vi "Motor Control Loop.vi"(8 "error in":errorcluster) -> (0 "error out":errorcluster)   [LabVIEW 2011]
uses:
  <vilib>/Simulation/Scripting/Companion Diagram/SimConfigNode/SimParams.ctl
  <vilib>/Simulation/Scripting/Companion Diagram/SimConfigNode/_simSolvers.ctl
  <vilib>/Simulation/Implementation/Shared/SIMSCR Execution Mode.ctl
  <vilib>/Platform/TimedLoop/XDataNode/timing_clust.ctl
  <vilib>/Platform/TimedLoop/XDataNode/nitl_modes.ctl
  <vilib>/Platform/TimedLoop/XDataNode/wakeup.ctl
  <vilib>/Simulation/Param Hierarchy/Typedefs/SIMPH Param Control Actions.ctl
  <vilib>/Simulation/Implementation/Shared/SIM limit type.ctl
  <vilib>/Simulation/Implementation/Shared/NILVSim_FinishedLate.vi
  <vilib>/Simulation/Utility/Implementation/SIM Halt.vi
  <vilib>/Simulation/Nonlinear/Implementation/NILVSim Saturation.llb/SIM Saturation (vector).vi
  <vilib>/Simulation/Nonlinear/Implementation/NILVSim Saturation.llb/SIM Saturation (scalar).vi
  <vilib>/Simulation/ContinuousLinear/Implementation/NILVSim Integrator new.llb/SIM Integrator distributor (scalar).vi
  <vilib>/Simulation/ContinuousLinear/Implementation/NILVSim Integrator new.llb/SIM Integrator collector (scalar).vi
  <vilib>/Simulation/ContinuousLinear/Implementation/NILVSim Integrator new.llb/SIM Integrator Collector (vector).vi
  <vilib>/Simulation/ContinuousLinear/Implementation/NILVSim Integrator new.llb/SIM Integrator Distributor (vector).vi
  <vilib>/Simulation/Implementation/Shared/SIM Is Init or Final Stage.vi
  <vilib>/Simulation/Implementation/Shared/NILVSim_Manager.vi
  <vilib>/Simulation/Implementation/Shared/NILVSim_ParamChanged.vi
  <vilib>/Simulation/Implementation/Shared/NILVSim_FinalizeModel.vi
  Robot Parameters/Robot Parameters.vi
  Roboteq/Public/Set RPM.vi
  <vilib>/Simulation/Implementation/Shared/SIM Unbundle Sim Info.vi
  <vilib>/Simulation/Implementation/Shared/NILVSim_GetModelError.vi
  <vilib>/Simulation/Implementation/Shared/SIM Bundle Sim Info.vi
  <vilib>/Simulation/Implementation/Shared/NILVSim_Initialize.vi
  <vilib>/robotics/Steering/Steering Frame/Apply Velocity to Motors.vi
  <vilib>/robotics/Steering/Steering Frame/Apply Steering Frame Velocity to Motors.vi
  Unsaturate Commanded Motor Velocities.vi
  <vilib>/robotics/Steering/Steering Frame/Get Velocity from Motors.vi
  <vilib>/robotics/Steering/Steering Frame/Get Steering Frame Velocity from Motors.vi
  <vilib>/Analysis/coordinate.llb/2D Cartesian Coordinate Rotation.vi
  <vilib>/Analysis/coordinate.llb/2D Cartesian Coordinate Rotation (Scalar).vi
  <vilib>/Simulation/Scripting/Companion Diagram/SimConfigNode/SimDog.xnode
  <vilib>/Platform/TimedLoop/XDataNode/XDataNode.xnode
  <vilib>/Simulation/Model Libraries/PID/SIM PID (Parallel).vi
  <vilib>/Simulation/Model Libraries/PID/SIM PID.vi
  <vilib>/Simulation/Implementation/XNodeFramework/SimXNode/SimX.xnode
  <vilib>/Platform/TimedLoop/XDataNode/XDNodeRunTimeDep.lvlib
  Roboteq/Roboteq.lvlib
  <vilib>/robotics/Steering/Steering Frame/NI_Robotics_Steering Frame.lvclass
  <vilib>/Analysis/NI_AALPro.lvlib
  <vilib>/Simulation/ContinuousLinear/Implementation/NILVSim Integrator new.llb/SIM Integrator (vector).vi
  <vilib>/Simulation/ContinuousLinear/Implementation/NILVSim Integrator new.llb/SIM Integrator (scalar).vi
  <vilib>/robotics/Utilities/NI_Robotics Utilities.lvlib
  <vilib>/Simulation/Implementation/Shared/NI_SIM_Implementation.lvlib
panel:
  out "Telemetry":T1={"Voltage"={0.0, 0.0, 0.0}, "Encoder Speed"={0, 0}, "Temps"={"IC Temp (C)"=0, "Ch1 Temp (C)"=0, "Ch2 Temp (C)"=0}, "Current"={0.0, 0.0, 0.0, 4.6238981750249924e+36}} {"Current" scale=0.0..16.0; "Temps"."IC Temp (C)" scale=0.0..150.0; "Temps"."Ch1 Temp (C)" scale=0.0..150.0; "Temps"."Ch2 Temp (C)" scale=0.0..150.0; "Encoder Speed" scale=-100.0..100.0; "Voltage" scale=8.0..14.0}
  in  "VISA resource name":refnum<visa-resource-name>
  in  "Debug":bool
  out "Command to Serial":string
  in  "End Loop":bool
  in  "stop?":bool
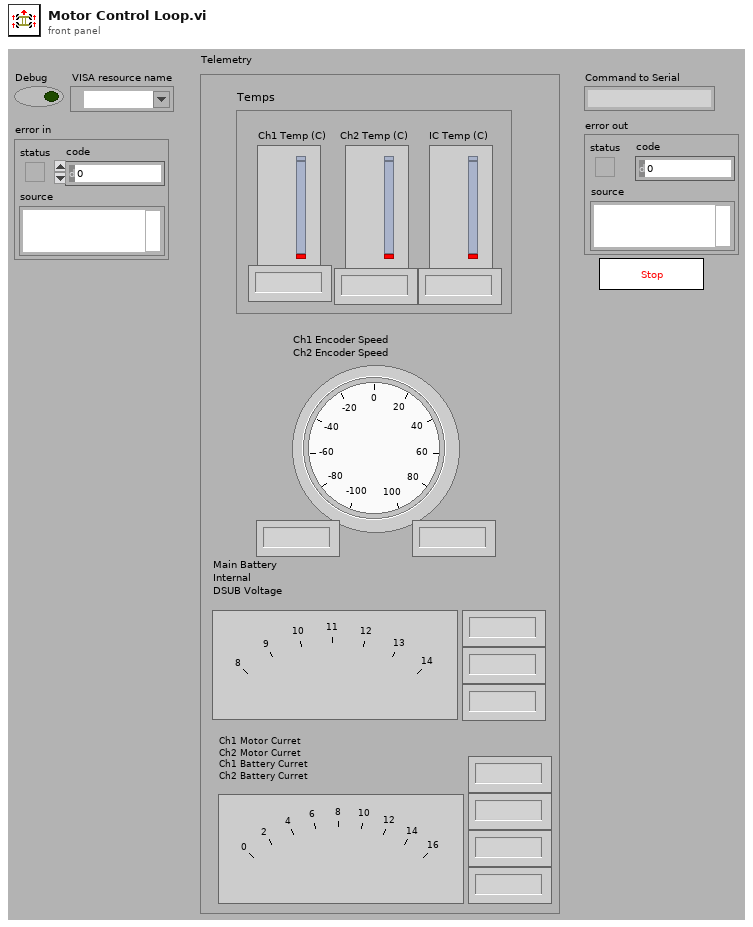
[diagram p1: front panel]
types:
  T1 = cluster{"Voltage":cluster{sgl, sgl, sgl}, "Encoder Speed":cluster{i32, i32}, "Temps":cluster{"IC Temp (C)":i32, "Ch1 Temp (C)":i32, "Ch2 Temp (C)":i32}, "Current":cluster{dbl, dbl, dbl, dbl}}
  T2 = typedef "SIMPH Param Control Actions.ctl" = enum16{"get params", "set params"}
  T3 = typedef "SIM limit type.ctl" = enum16{"upper", "lower", "both", "none"}
  T4 = typedef "XDNodeRunTimeDep.lvlib/timing_clust.ctl" = cluster{"Expected End [f-1]":u64, "Actual End [f-1]":u64, "Finished Late? [f-1]":bool, "Expected End [i-1]":u64, "Actual End [i-1]":u64, "Finished Late? [i-1]":bool, "Expected Start [i]":u64, "Actual Start [i]":u64, "Expected Start [f]":u64, "Actual Start [f]":u64, "Source Name":string, "Structure Name":string, "Period":i64, "Deadline":i64, "Offset":i64, "Start":i64, "Priority":i32, "Timeout":i32, "Mode":T5, "Wakeup Reason":T6, "Error":errorcluster, "Source Type":string, "Secondary Source Type":string, "Global End Time":u64, "Global Start Time":u64, "Frame Duration":u64, "Iteration Duration":u64, "Assigned CPU":i32, "I/O Scan Engine Mode":u32}
  T5 = typedef "XDNodeRunTimeDep.lvlib/nitl_modes.ctl" = enum32{"No Change", "Process missed periods, maintain original phase", "Discard missed periods, maintain original phase", "Process missed periods, ignore original phase", "Discard missed periods, ignore original phase"}
  T6 = typedef "XDNodeRunTimeDep.lvlib/wakeup.ctl" = enum32{"Normal", "Aborted", "Asynchronous wakeup", "Timing source error", "Timed loop error", "Timeout"}
  T7 = typedef "SimParams.ctl" = cluster{"Initial Time (s)":dbl, "Final Time (s)":dbl, "Step Size (s)":dbl, "ODE Solver":T8, "Minimum Step Size (s)":dbl, "Maximum Step Size (s)":dbl, "Relative Tolerance":dbl, "Absolute Tolerance":dbl, "Software Timing":bool, "Initial Step Size (s)":dbl, "Automatic Fixed Step Size?":bool, "Automatic Discrete Step Size?":bool, "Discrete Step Size (s)":dbl, "Calculate using Time Step":bool, "Solver Wired?":bool, "Prev.Frm.Expected End":u64, "Prev.Frm.Actual End":u64, "Prev.Frm.Finished Late?":bool, "Prev.Iter.Expected End":u64, "Prev.Iter.Actual End":u64, "Prev.Iter.Finished Late?":bool, "Expected Iteration Start":u64, "Actual Iteration Start":u64, "Expected Frame Start":u64, "Actual Frame Start":u64, "Source Name":string, "Name":string, "Period":i64, "Deadline":i64, "Offset":i64, "Start":i64, "Priority":i32, "Timeout":i32, "Processor":i32, "Mode":enum32{"No Change", "Process missed periods, maintain original phase", "Discard missed periods, maintain original phase", "Process missed periods, ignore original phase", "Discard missed periods, ignore original phase"}, "Wakeup reason":enum32{"Normal", "Aborted", "Asynchronous wakeup", "Timing source error", "Timed loop error", "Timeout"}, "Error":errorcluster, "Source Type":string, "Secondary Source Type":string, "Global End Time":u64, "Global Start Time":u64, "Full Solver Reset":bool, "Execution Mode":T9, "Nan/Inf Check":bool, "Custom Solver Library":string, "Solver Is Variable":bool, "custom solver name":string}
  T8 = typedef "_simSolvers.ctl" = enum16{"Runge-Kutta 1 (Euler)", "Runge-Kutta 2", "Runge-Kutta 3", "Runge-Kutta 4", "Runge-Kutta 23 (variable)", "Runge-Kutta 45 (variable)", "BDF (variable)", "Adams-Moulton (variable)", "Rosenbrock (variable)", "Discrete States Only", "Linearizer", "State Query", "Trim Eval", "Custom Solver"}
  T9 = typedef "SIMSCR Execution Mode.ctl" = u16
  T10 = cluster{"main battery voltage (V)":sgl, "internal voltage (V)":sgl, "DSUB voltage (V)":sgl}
  T11 = cluster{" Ch1  Motor current (I)":sgl, " Ch2 Motor current (I)":sgl, " Ch1 Battery current (I)":sgl, " Ch2 Battery current (I)":sgl}
  T12 = cluster{"Ch1 Temp (C)":i32, "Ch2 Temp (C)":i32, "IC Temp (C)":i32}
  T13 = cluster{"Encoder Speed (RPM)":i32, "Encoder Speed (RPM)":i32}
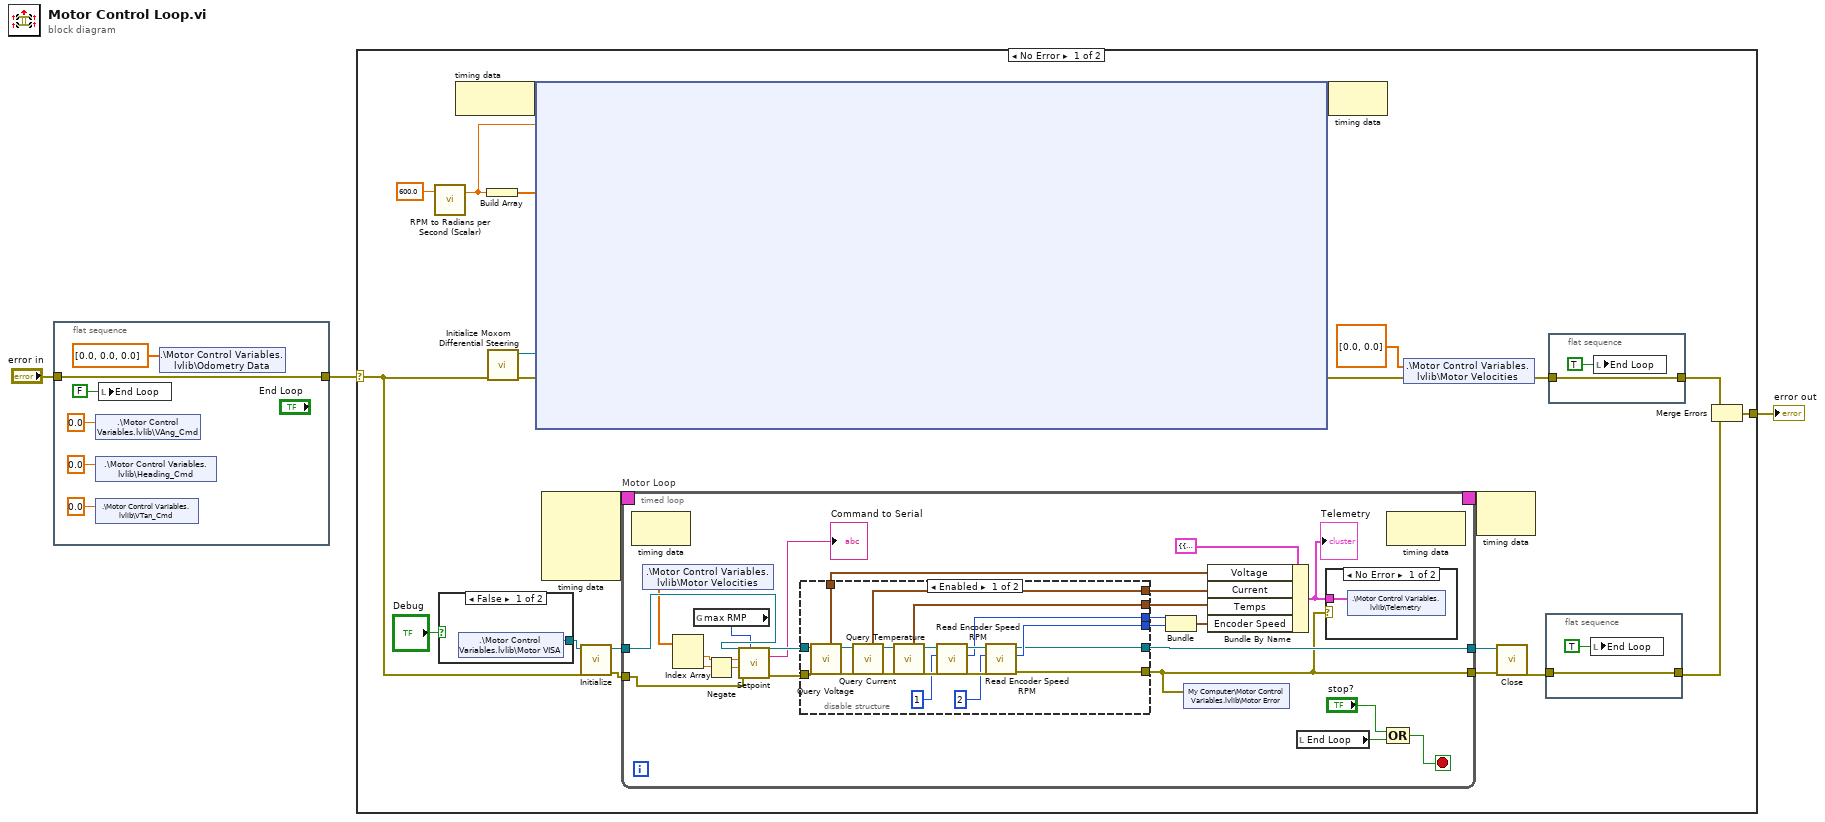
[diagram p0: block diagram]
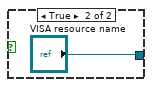
[diagram p2: hidden frame]
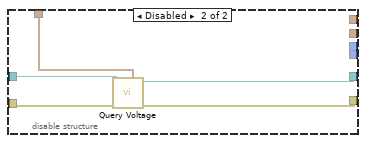
[diagram p3: hidden frame]
diagram:
  n1 = flat-sequence {
    tunnel: [w5] -> w2
    tunnel: "error in" -> [w5]
    frame #0 {
      n2 = shared-variable ".\\Motor Control Variables.lvlib\\VAng_Cmd"(0.0 ("VX_Cmd")) -> ()  [unwired: 1 in, 1 out]
      n3 = shared-variable ".\\Motor Control Variables.lvlib\\Heading_Cmd"(0.0 ("Heading_Cmd")) -> ()  [unwired: 1 in, 1 out]
      n4 = shared-variable ".\\Motor Control Variables.lvlib\\VTan_Cmd"(0.0 ("VY_Cmd")) -> ()  [unwired: 1 in, 1 out]
      n5 = local write "End Loop"(FALSE ("End Loop")) -> ()
      n6 = shared-variable ".\\Motor Control Variables.lvlib\\Odometry Data"(dbl[] [0.0, 0.0, 0.0] ("Odometry Data")) -> ()  [unwired: 1 in, 1 out]
    }
  }
  n7 = case shown="No Error" w2 {
    selector: w2 -> [w28 w495]
    tunnel: [w30 w495] -> w1
    frame No Error {
      n8 = call <vilib>:"RPM to Radians per Second (Scalar).vi"("rpm"=600.0 ("Numeric")) -> ("radians per second"=w16:dbl)  [unwired: 2 in]
      n9 = case shown="False" "Debug" {
        tunnel: [w33 "VISA resource name"] -> w29
        frame False {
          n10 = shared-variable ".\\Motor Control Variables.lvlib\\Motor VISA"() -> (w33:refnum<visa-resource-name>)  [unwired: 1 in, 1 out]
        }
        frame True {
        }
      }
      n11 = node-c288() -> (w18:variant)  [unwired: 1 in]
      n12 = Build Array(w16) -> (w15:dbl[])
      n13 = call "Initialize Moxom Differential Steering.vi"("error in (no error)"=w28) -> ("error out"=w12:errorcluster, "differential steering frame out"=w13:refnum<class "NI_Robotics_Differential Steering Frame.lvclass">)  [unwired: 9 in]
      n14 = node-c254 ("Simulation Loop 3")(w18, w16, w15, w12, w13) -> (w17:variant, w11:errorcluster)
      n15 = node-c288() -> (w20:T4)  [unwired: 4 in]
      n16 = call "Initialize.vi"("error in (no error)"=w28, "VISA resource name"=w29) -> ("error out"=w26:errorcluster, "VISA resource name out"=w27:refnum<visa-resource-name>)  [unwired: 8 in]
      n17 = timed-loop "Motor Loop" {
        tunnel: w27 -> [w459]
        tunnel: w26 -> [w458]
        tunnel: [w453] -> w25
        tunnel: [w454] -> w31
        timing: w20 -> [_]
        timing-out: [_] -> w19
        stop <- w460 stop-if-true
        n18 = node-c288() -> ()  [unwired: 1 in, 1 out]
        n19 = shared-variable ".\\Motor Control Variables.lvlib\\Motor Velocities"() -> (w441:dbl[])  [unwired: 1 in, 1 out]
        n20 = Index Array(array=w441) -> (element #1=w449:dbl, element #2=w442:dbl)  [unwired: 2 in]
        n21 = global read "Robot Parameters.vi" "max RMP"() -> (w450:i32)
        n22 = Negate(x=w442) -> (-x=w439:dbl)
        n23 = call-poly "Setpoint.vi"("Max RPM"=w450, "error in (no error)"=w458, "Motor2 Speed (RPM)"=w439, "Motor1 Speed (RPM)"=w449, "VISA resource name"=w459) -> ("error out"=w455:errorcluster, "Command"=→"Command to Serial":string, "VISA resource name out"=w456:refnum<visa-resource-name>)  [unwired: 4 in]
        n24 = disable-structure shown="Enabled" {
          disable-tunnel: w456 -> [w480 w485]
          disable-tunnel: w455 -> [w479 w484]
          disable-tunnel: [w474 _] -> w445
          disable-tunnel: [w473 _] -> w444
          disable-tunnel: [w463 w483] -> w454
          disable-tunnel: [w472 _] -> w446
          disable-tunnel: [w462 w482] -> w453
          disable-tunnel: [w471 w481] -> w447
          disable-tunnel: [w466 _] -> w440
          frame Enabled {
            n25 = call "Query Voltage.vi"("error in (no error)"=w479, "VISA resource name"=w480) -> ("error out"=w469:errorcluster, "VISA resource name out"=w470:refnum<visa-resource-name>, "Voltages"=w471:T10)  [unwired: 4 in, 3 out]
            n26 = call "Query Current.vi"("error in (no error)"=w469, "VISA resource name"=w470) -> ("error out"=w467:errorcluster, "VISA resource name out"=w468:refnum<visa-resource-name>, "Motor Currents"=w466:T11)  [unwired: 3 in, 4 out]
            n27 = call "Query Temperature.vi"("error in (no error)"=w467, "VISA resource name"=w468) -> ("error out"=w477:errorcluster, "VISA resource name out"=w478:refnum<visa-resource-name>, "Temps"=w472:T12)  [unwired: 4 in, 3 out]
            n28 = call "Read Encoder Speed RPM.vi"("error in (no error)"=w477, "channel number"=u8 1, "VISA resource name"=w478) -> ("error out"=w475:errorcluster, "Encoder Speed (RPM)"=w474:i32, "VISA resource name out"=w476:refnum<visa-resource-name>)  [unwired: 6 in]
            n29 = call "Read Encoder Speed RPM.vi"("error in (no error)"=w475, "channel number"=u8 2, "VISA resource name"=w476) -> ("error out"=w462:errorcluster, "Encoder Speed (RPM)"=w473:i32, "VISA resource name out"=w463:refnum<visa-resource-name>)  [unwired: 6 in]
          }
          frame Disabled {
            n30 = call "Query Voltage.vi"("error in (no error)"=w484, "VISA resource name"=w485) -> ("error out"=w482:errorcluster, "VISA resource name out"=w483:refnum<visa-resource-name>, "Voltages"=w481:T10)  [unwired: 4 in, 3 out]
          }
        }
        n31 = Bundle("Encoder Speed (RPM)"=w445, "Encoder Speed (RPM)"=w444) -> (w443:T13)  [unwired: 1 in]
        n32 = shared-variable "My Computer\\Motor Control Variables.lvlib\\Motor Error"(w453) -> ()  [unwired: 1 in, 1 out]
        n33 = Bundle By Name(cluster=T1 {"Voltage"={0.0, 0.0, 0.0}, "Encoder Speed"={0, 0}, "Temps"={"IC Temp (C)"=0, "Ch1 Temp (C)"=0, "Ch2 Temp (C)"=0}, "Current"={0.0, 0.0, 0.0, 0.0}} ("Telemetry"), "Voltage"=w447, "Current"=w440, "Temps"=w446, "Encoder Speed"=w443) -> (w451:T1)
        "Telemetry" <- w451
        n34 = local read "End Loop"() -> (w457:bool)
        n35 = case shown="No Error" w453 {
          tunnel: w451 -> [w488 _]
          frame No Error {
            n36 = shared-variable ".\\Motor Control Variables.lvlib\\Telemetry"(w488) -> ()  [unwired: 1 in, 1 out]
          }
          frame Error {
          }
        }
        n37 = node-c288() -> ()  [unwired: 1 in, 1 out]
        n38 = Compound Arithmetic op=OR("stop?", w457) -> (w460:bool)
      }
      n39 = node-c288(w17) -> ()  [unwired: 1 out]
      n40 = shared-variable ".\\Motor Control Variables.lvlib\\Motor Velocities"(dbl[] [0.0, 0.0] ("Motor Velocities"), error in=w11) -> (error out=w21:errorcluster)
      n41 = node-c288(w19) -> ()  [unwired: 1 out]
      n42 = call "Close.vi"("error in (no error)"=w25, "VISA resource name"=w31) -> ("error out"=w24:errorcluster)  [unwired: 9 in]
      n43 = flat-sequence {
        tunnel: w24 -> [w491]
        tunnel: [w491] -> w23
        frame #0 {
          n44 = local write "End Loop"(TRUE ("End Loop")) -> ()
        }
      }
      n45 = flat-sequence {
        tunnel: [w493] -> w22
        tunnel: w21 -> [w493]
        frame #0 {
          n46 = local write "End Loop"(TRUE ("End Loop")) -> ()
        }
      }
      n47 = Merge Errors(w22, w23) -> (w30:errorcluster)
    }
    frame Error {
    }
  }
  "error out" <- w1
